vi "test_crc32.vi"() -> (3 "All Passed?":bool)   [LabVIEW 2021]
uses:
  src/hashlib.lvlib
panel:
  in  "Data in":string="123456789"
  out "CRC-32 out":T1(array[cluster]) {"CRC-32" format="%08x"}
  in  "CRC-32 Types":T2(array[cluster])=[{"Name"="CRC-32", "CRC-32"=3421780262, "Initial"=4294967295, "Poly"=79764919, "XorOut"=4294967295, "ReflectIn"=TRUE, "ReflectOut"=TRUE}, {"Name"="CRC-32/BZIP2", "CRC-32"=4236843288, "Initial"=4294967295, "Poly"=79764919, "XorOut"=4294967295, "ReflectIn"=FALSE, "ReflectOut"=FALSE}, {"Name"="CRC-32C", "CRC-32"=3808858755, "Initial"=4294967295, "Poly"=517762881, "XorOut"=4294967295, "ReflectIn"=TRUE, "ReflectOut"=TRUE}, {"Name"="CRC-32D", "CRC-32"=2268157302, "Initial"=4294967295, "Poly"=2821953579, "XorOut"=4294967295, "ReflectIn"=TRUE, "ReflectOut"=TRUE}, {"Name"="CRC-32/JAMCRC", "CRC-32"=873187033, "Initial"=4294967295, "Poly"=79764919, "XorOut"=0, "ReflectIn"=TRUE, "ReflectOut"=TRUE}, {"Name"="CRC-32/MPEG-2", "CRC-32"=58124007, "Initial"=4294967295, "Poly"=79764919, "XorOut"=0, "ReflectIn"=FALSE, "ReflectOut"=FALSE}, {"Name"="CRC-32/POSIX", "CRC-32"=1985902208, "Initial"=0, "Poly"=79764919, "XorOut"=4294967295, "ReflectIn"=FALSE, "ReflectOut"=FALSE}, {"Name"="CRC-32Q", "CRC-32"=806403967, "Initial"=0, "Poly"=2168537515, "XorOut"=0, "ReflectIn"=FALSE, "ReflectOut"=FALSE}, {"Name"="CRC-32/XFER", "CRC-32"=3171672888, "Initial"=0, "Poly"=175, "XorOut"=0, "ReflectIn"=FALSE, "ReflectOut"=FALSE}] {"XorOut" format="%08x"; "CRC-32" format="%08x"; "Poly" format="%08x"; "Initial" format="%08x"}
  # "https://crccalc.com/"
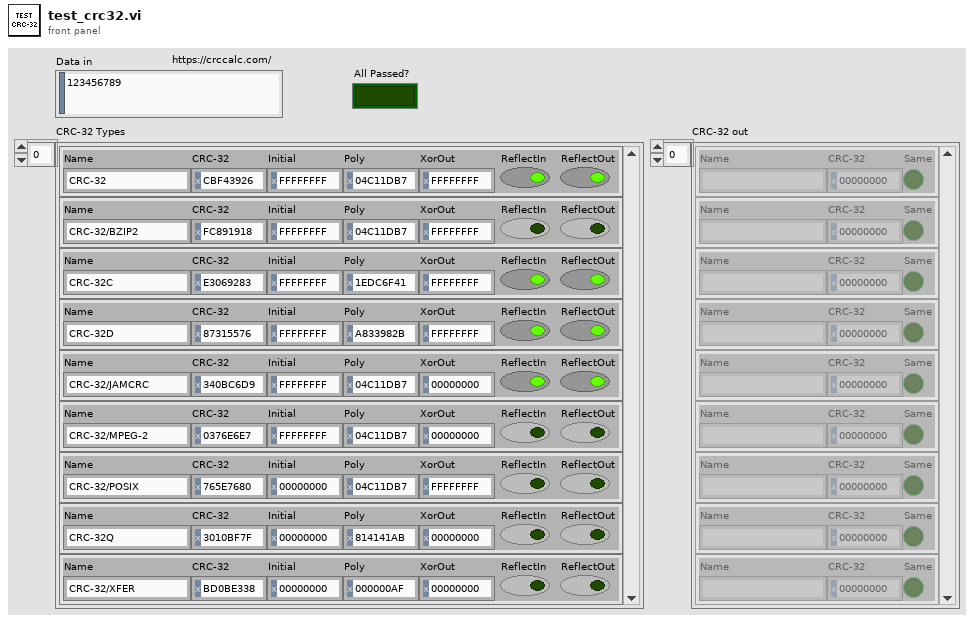
[diagram p1: front panel]
types:
  T1 = cluster{"Name":string, "CRC-32":u32, "Same":bool}[]
  T2 = cluster{"Name":string, "CRC-32":u32, "Initial":u32, "Poly":u32, "XorOut":u32, "ReflectIn":bool, "ReflectOut":bool}[]
  T3 = cluster{"Name":string, "CRC-32":u32, "Same":bool}
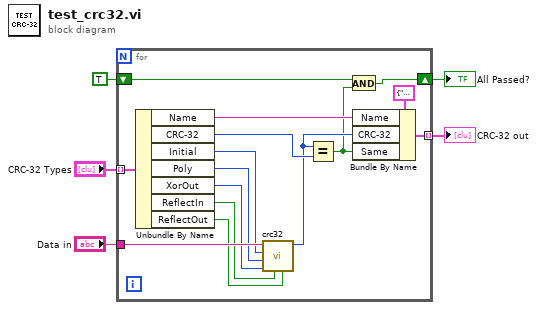
[diagram p0: block diagram]
diagram:
  n1 = for {
    tunnel: "Data in" -> [w20]
    tunnel: "CRC-32 Types" -> [w19] mode=indexing
    tunnel: [w17] -> w3 mode=indexing
    shift-right: [w12] -> w1
    shift-left: TRUE -> [w14]
    n2 = Unbundle By Name(w19) -> ("Name"=w18:string, "CRC-32"=w16:u32, "Initial"=w11:u32, "Poly"=w10:u32, "XorOut"=w9:u32, "ReflectIn"=w8:bool, "ReflectOut"=w7:bool)
    n3 = call "crc32.vi"("Reflect Output? (T)"=w7, "Reflect Input? (T)"=w8, "Xor Out (0xFFFFFFFF)"=w9, "Poly (0x04C11DB7)"=w10, "Init (0xFFFFFFFF)"=w11, "Data in"=w20) -> ("CRC-32"=w15:u32)  [unwired: 5 in]
    n4 = Equal?(x=w15, y=w16) -> (x = y?=w13:bool)
    n5 = And(x=w14, y=w13) -> (x .and. y?=w12:bool)
    n6 = Bundle By Name(cluster=T3 {"Name"="", "CRC-32"=0, "Same"=FALSE} ("CRC-16"), "Name"=w18, "CRC-32"=w15, "Same"=w13) -> (w17:T3)
  }
  "CRC-32 out" <- w3
  "All Passed?" <- w1
